vi "Spaghetti.vi"() -> ()   [LabVIEW 2020]
uses:
  controls/StateMachineVariables.ctl
  <vilib>/vision/Avi.llb/IMAQ AVI2 Refnum.ctl
  <vilib>/userDefined/High Color/IMAQdx.ctl
  <vilib>/vision/Deep Learning.llb/IMAQ DL Model Refnum.ctl
  <vilib>/vision/Image Controls.llb/IMAQ Image.ctl
panel:
  in  "Cluster":T1
  in  "Turn on the replay mode":bool=TRUE
  out "Replay mode":bool
  in  "?":T6(tab)
  in  "Camera Name":refnum<k21> caption="IMAQdx Session"
  out "fps cam":dbl
  out "height":u32
  out "width":u32
  in  "Start Frame Number":u32
  out "Actual frame":u32
  in  "Frame increment":i32=1
  in  "Video fps":u32=30
  in  "Video filename":string="test_moving2.avi"
  in  "Height":i32=1080
  in  "Width":i32=1920
  out "fps detection":dbl
  out "Distance":sgl(graph)
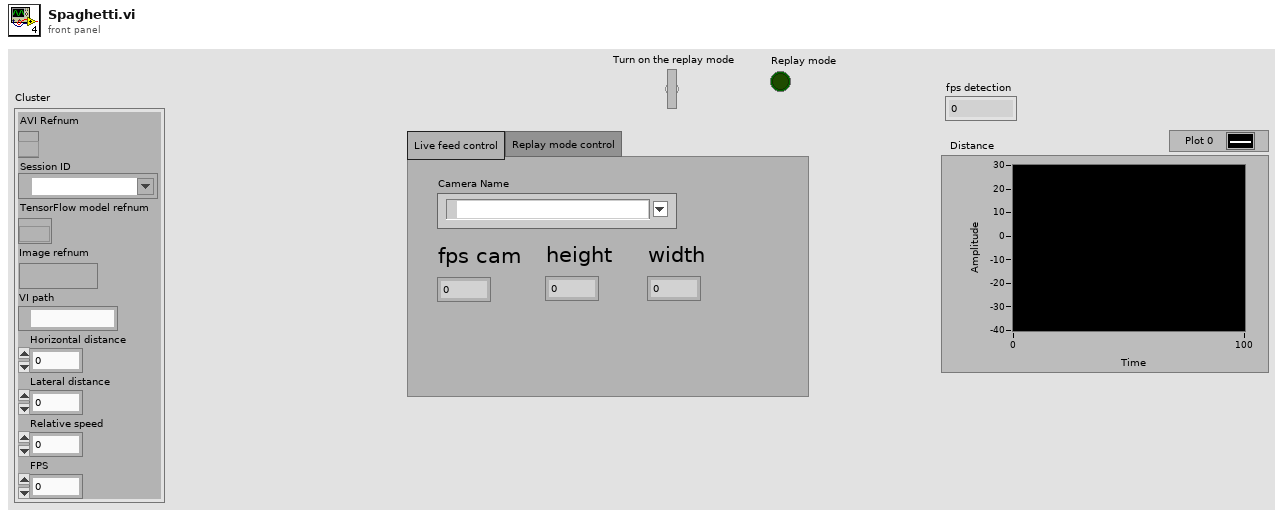
[diagram p1: front panel]
types:
  T1 = typedef "StateMachineVariables.ctl" = cluster{"AVI Refnum":T2, "Session ID":T3, "TensorFlow model refnum":T4, "Image refnum":T5, "VI path":path, "Horizontal distance":dbl, "Lateral distance":dbl, "Relative speed":dbl, "FPS":dbl}
  T2 = typedef "IMAQ AVI2 Refnum.ctl" = refnum<k20>
  T3 = typedef "IMAQdx.ctl" = refnum<k21>
  T4 = typedef "IMAQ DL Model Refnum.ctl" = refnum<k20>
  T5 = typedef "IMAQ Image.ctl" = refnum<image>
  T6 = enum32{"Live feed control", "Replay mode control"}
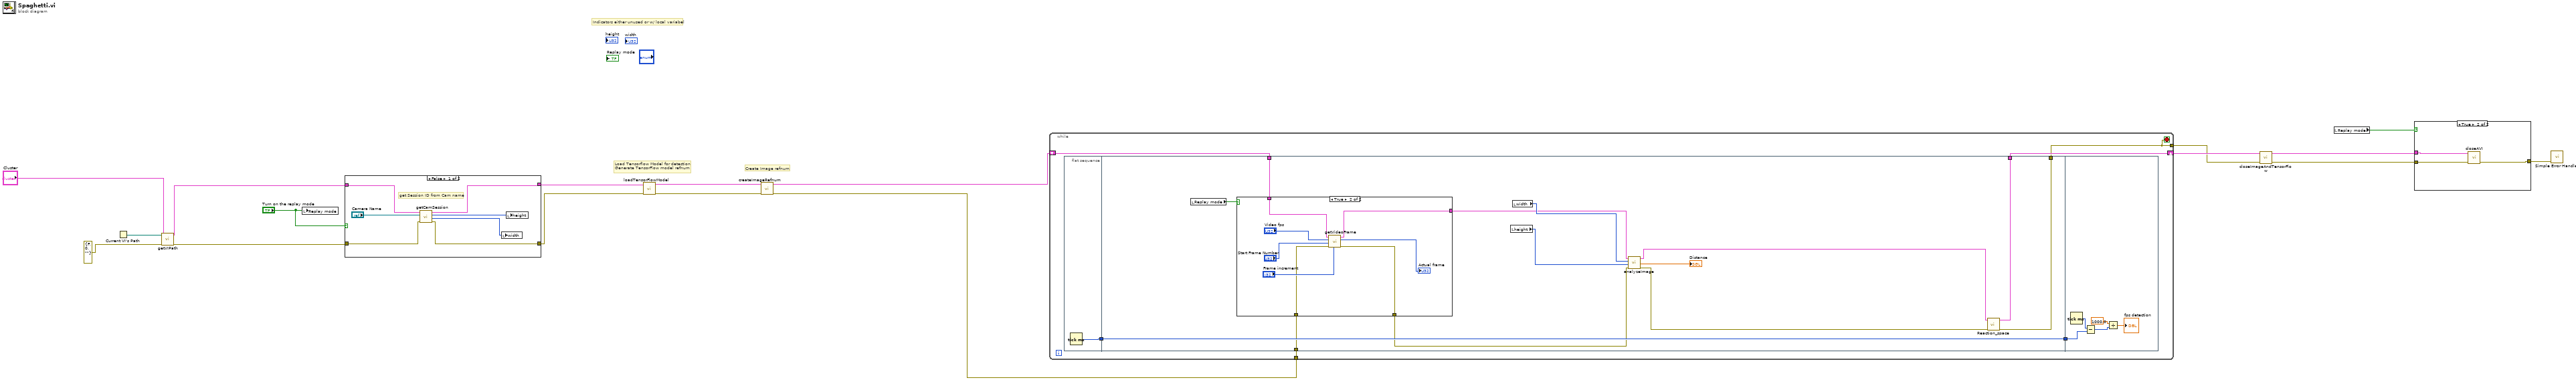
[diagram p0: block diagram]
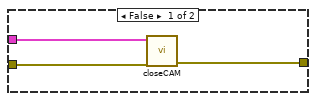
[diagram p2: hidden frame]
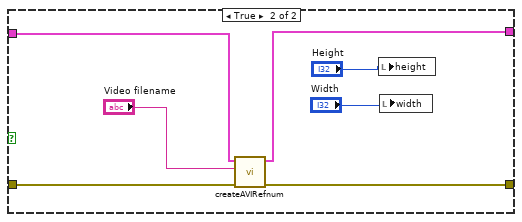
[diagram p3: hidden frame]
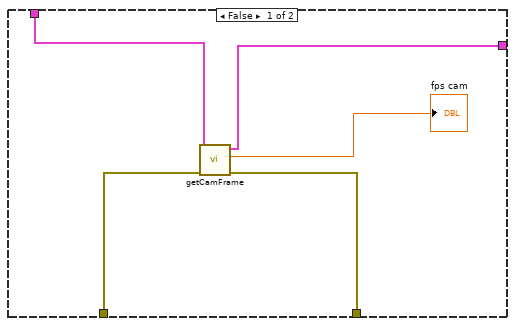
[diagram p4: hidden frame]
diagram:
  # "Create Image refnum"
  # "Indicators either unused or w/ local variabel"
  # "Load Tensorflow Model for detection\nGenerate TensorFlow model refnum"
  n1 = Current VI's Path() -> (path=w10:path)
  n2 = call "getVIPath.vi"("error in"=errorcluster {"status"=FALSE, "code"=0, "source"=""} ("error constant"), "Cluster in"="Cluster", "path"=w10) -> ("error out"=w2:errorcluster, "Cluster out"=w8:T1)  [unwired: 7 in]
  n3 = local write "Replay mode"("Turn on the replay mode") -> ()
  n4 = case shown="False" "Turn on the replay mode" {
    tunnel: [w21 w29] -> w7
    tunnel: w8 -> [w22 w28]
    tunnel: [w20 w27] -> w3
    tunnel: w2 -> [w19 w26]
    frame False {
      # "get Session ID from Cam name"
      n5 = call "getCamSession.vi"("error in"=w19, "Camera name"="Camera Name", "Input cluster"=w22) -> ("error out"=w20:errorcluster, "Width"=w25:u32, "Height"=w24:u32, "Output cluster"=w21:T1)  [unwired: 5 in]
      n6 = local write "width"(w25) -> ()
      n7 = local write "height"(w24) -> ()
    }
    frame True {
      n8 = call "createAVIRefnum.vi"("error in"=w26, "Video filename"="Video filename", "Input cluster"=w28) -> ("error out"=w27:errorcluster, "Output cluster"=w29:T1)  [unwired: 7 in]
      n9 = local write "height"("Height") -> ()
      n10 = local write "width"("Width") -> ()
    }
  }
  n11 = call "loadTensorFlowModel.vi"("error in"=w3, "Input cluster"=w7) -> ("error out"=w4:errorcluster, "Output cluster"=w6:T1)  [unwired: 8 in]
  n12 = call "createImageRefnum.vi"("error in"=w4, "Output cluster in"=w6) -> ("error out"=w5:errorcluster, "Output cluster out"=w14:T1)  [unwired: 8 in]
  n13 = while {
    shift-right: [w34] -> w12
    shift-left: w14 -> [w36]
    tunnel: w5 -> [w35]
    tunnel: [w33] -> w11
    stop <- w33 stop-if-true
    n14 = flat-sequence {
      tunnel: [w39] -> w38
      tunnel: w38 -> [w52]
      tunnel: [w52] -> w37
      tunnel: w36 -> [w50]
      tunnel: w35 -> [w49]
      tunnel: [w48] -> w33
      tunnel: [w47] -> w34
      tunnel: w37 -> [w69]
      frame #0 {
        n15 = Tick Count (ms)() -> (millisecond timer value=w39:u32)
      }
      frame #1 {
        n16 = local read "Replay mode"() -> (w51:bool)
        n17 = case shown="True" w51 {
          tunnel: [w55 w63] -> w41
          tunnel: w50 -> [w57 w59]
          tunnel: w49 -> [w54 w62]
          tunnel: [w53 w58] -> w44
          frame False {
            n18 = call "getCamFrame.vi"("error in (no error)"=w54, "Cluster"=w57) -> ("error out"=w55:errorcluster, "Acquired Frames per Second"=→"fps cam":dbl, "output cluster"=w53:T1)  [unwired: 7 in]
          }
          frame True {
            n19 = call "getVideoFrame.vi"("Frame increment"="Frame increment", "error in (no error)"=w62, "Start Frame Number"="Start Frame Number", "Video fps"="Video fps", "Input cluster"=w59) -> ("error out"=w63:errorcluster, "Actual frame"=→"Actual frame":u32, "Output cluster"=w58:T1)  [unwired: 4 in]
          }
        }
        n20 = local read "height"() -> (w42:u32)
        n21 = local read "width"() -> (w45:u32)
        n22 = call "analyzeImage.vi"("error in"=w41, "Height"=w42, "Width"=w45, "Input cluster"=w44) -> ("error out"=w40:errorcluster, "Output cluster"=w43:T1, "Distance"=→"Distance":sgl)  [unwired: 3 in, 2 out]
        n23 = call "Reaction_space.vi"("error in"=w40, "Input cluster"=w43) -> ("error out"=w48:errorcluster, "Ouptut cluster"=w47:T1)  [unwired: 8 in]
      }
      frame #2 {
        n24 = Tick Count (ms)() -> (millisecond timer value=w70:u32)
        n25 = Subtract(x=w70, y=w69) -> (x-y=w67:u32)
        n26 = Divide(x=1000.0, y=w67) -> (x/y=→"fps detection":dbl)
      }
    }
  }
  n27 = call "closeImageAndTensorFlow.vi"("error in (no error)"=w11, "Input cluster"=w12) -> ("error out"=w18:errorcluster, "Output cluster"=w13:T1)  [unwired: 8 in]
  n28 = local read "Replay mode"() -> (w16:bool)
  n29 = case shown="True" w16 {
    tunnel: w18 -> [w73 w76]
    tunnel: [w72 w75] -> w17
    tunnel: w13 -> [w71 w74]
    frame False {
      n30 = call "closeCAM.vi"("error in (no error)"=w73, "Input cluster"=w71) -> ("error out"=w72:errorcluster)  [unwired: 8 in, 1 out]
    }
    frame True {
      n31 = call "closeAVI.vi"("error in (no error)"=w76, "Input cluster"=w74) -> ("error out"=w75:errorcluster)  [unwired: 8 in, 1 out]
    }
  }
  n32 = call <vilib>:"Simple Error Handler.vi"("error in (no error)"=w17) -> ()  [unwired: 4 in, 5 out]
